vi "for loop 9.vi"() -> ()   [LabVIEW 2025]
panel:
  in  "Numeric 2":dbl
  out "Numeric":dbl
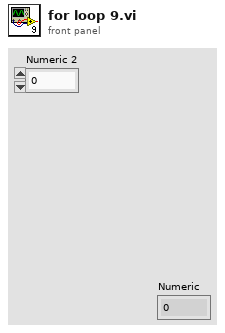
[diagram p1: front panel]
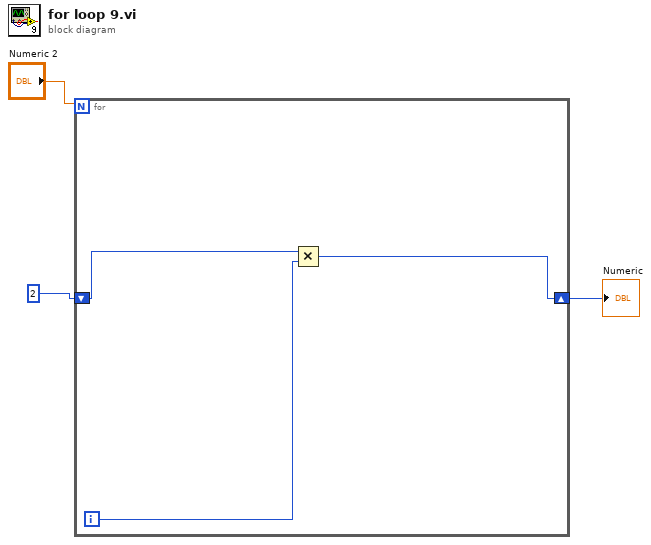
[diagram p0: block diagram]
diagram:
  n1 = for {
    N: "Numeric 2" -> [_]
    shift-right: [w4] -> w2
    shift-left: 2 -> [w5]
    i -> [w6]
    n2 = Multiply(x=w5, y=w6) -> (x*y=w4:i32)
  }
  "Numeric" <- w2
